vi "Reading buffer.vi"(3 "错误输入":errorcluster, 4 "Options":string(combo), 5 "缓冲区名称":string(combo), 6 "VISA资源名称":refnum<visa-resource-name>) -> (0 "错误输出":errorcluster, 1 "缓冲区数据":dbl[](array[numeric]), 2 "VISA资源名称输出":refnum<visa-resource-name>)   [LabVIEW 2020]
panel:
  out "结果字符串":string
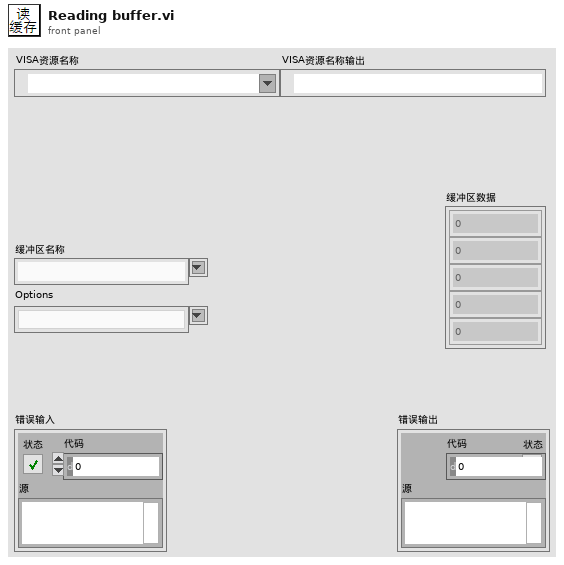
[diagram p1: front panel]
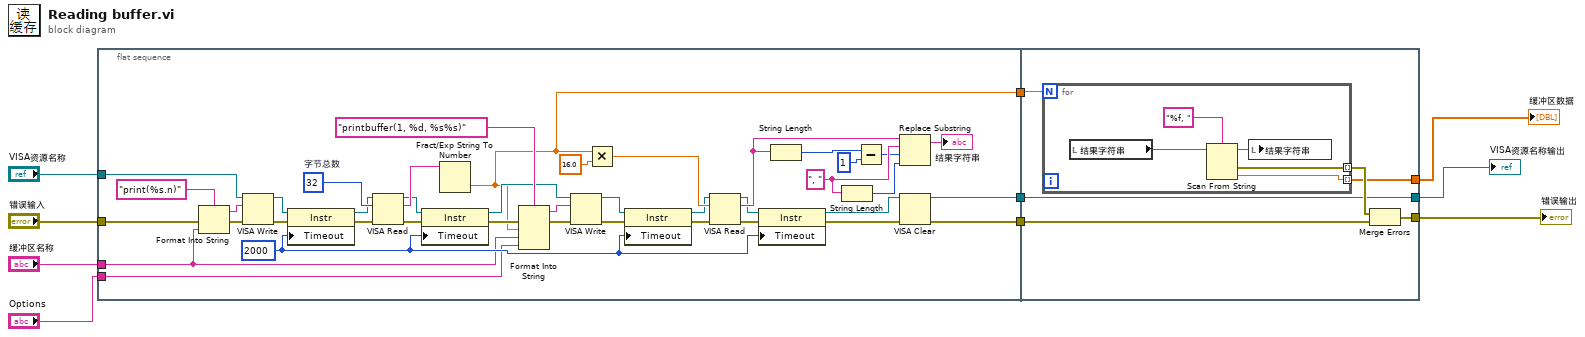
[diagram p0: block diagram]
diagram:
  n1 = flat-sequence {
    tunnel: "错误输入" -> [w49]
    tunnel: "缓冲区名称" -> [w17]
    tunnel: "VISA资源名称" -> [w48]
    tunnel: [w18] -> w8
    tunnel: [w12] -> w7
    tunnel: [w13] -> w6
    tunnel: "Options" -> [w16]
    tunnel: [w56] -> w1
    tunnel: w8 -> [w57]
    tunnel: w7 -> [w55]
    tunnel: w6 -> [w53]
    tunnel: [w53] -> w5
    tunnel: [w52] -> w4
    frame #0 {
      w19 = u32 2000 ("General Settings:Timeout Value")
      w41 = ", "
      w45 = u32 32  # 字节总数
      n2 = Format Into String(format string="print(%s.n)" ("格式字符串"), error in=w49, w17) -> (resulting string=w46:string, error out=w47:errorcluster)  [unwired: 1 in]
      n3 = VISA Write(VISA resource name=w48, write buffer=w46, error in (no error)=w47) -> (VISA resource name out=w30:refnum<visa-resource-name>, error out=w29:errorcluster)  [unwired: 1 out]
      n4 = property class="Instr"(reference=w30, error in=w29, "Timeout"=w19) -> (reference out=w32:refnum<visa-resource-name>, error out=w31:errorcluster)
      n5 = VISA Read(VISA resource name=w32, byte count=w45, error in (no error)=w31) -> (VISA resource name out=w27:refnum<visa-resource-name>, read buffer=w44:string, error out=w28:errorcluster)  [unwired: 1 out]
      n6 = property class="Instr"(reference=w27, error in=w28, "Timeout"=w19) -> (reference out=w26:refnum<visa-resource-name>, error out=w25:errorcluster)
      n7 = Fract/Exp String To Number(string=w44) -> (number=w18:dbl)  [unwired: 3 in, 1 out]
      n8 = Format Into String(format string="printbuffer(1, %d, %s%s)" ("格式字符串"), error in=w25, w18, w17, w16) -> (resulting string=w43:string, error out=w42:errorcluster)  [unwired: 1 in]
      n9 = VISA Write(VISA resource name=w26, write buffer=w43, error in (no error)=w42) -> (VISA resource name out=w24:refnum<visa-resource-name>, error out=w23:errorcluster)  [unwired: 1 out]
      n10 = Multiply(x=w18, y=16.0) -> (x*y=w33:dbl)
      n11 = property class="Instr"(reference=w24, error in=w23, "Timeout"=w19) -> (reference out=w21:refnum<visa-resource-name>, error out=w22:errorcluster)
      n12 = VISA Read(VISA resource name=w21, byte count=w33, error in (no error)=w22) -> (VISA resource name out=w20:refnum<visa-resource-name>, read buffer=w36:string, error out=w15:errorcluster)  [unwired: 1 out]
      n13 = property class="Instr"(reference=w20, error in=w15, "Timeout"=w19) -> (reference out=w14:refnum<visa-resource-name>, error out=w11:errorcluster)
      n14 = String Length(string=w36) -> (length=w38:i32)
      n15 = String Length(string=w41) -> (length=w40:i32)
      n16 = Subtract(x=w38, y=1) -> (x-y=w39:i32)
      n17 = Replace Substring(2:w40, 3:w39, 4:w41, 5:w36) -> (1:→"结果字符串":string)  [unwired: 1 out]
      n18 = VISA Clear(VISA resource name=w14, error in (no error)=w11) -> (VISA resource name out=w13:refnum<visa-resource-name>, error out=w12:errorcluster)
    }
    frame #1 {
      n19 = for {
        N: w57 -> [_]
        tunnel: [w61] -> w52 mode=indexing
        tunnel: [w58] -> w54 mode=indexing
        n20 = local read "结果字符串"() -> (w60:string)
        n21 = Scan From String(format string="%f, " ("格式字符串"), input string=w60) -> (remaining string=w59:string, error out=w58:errorcluster, output 1=w61:dbl)  [unwired: 3 in, 1 out]
        n22 = local write "结果字符串"(w59) -> ()
      }
      n23 = Merge Errors(w54, w55) -> (w56:errorcluster)
    }
  }
  "VISA资源名称输出" <- w5
  "缓冲区数据" <- w4
  "错误输出" <- w1
